vi "PKYK_TRAIL_TOKEN.vi"(1 "RFID In":string) -> (0 "PKYK?TRAIL":string)   [LabVIEW 2020]
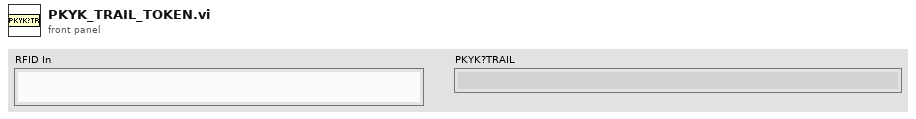
[diagram p1: front panel]
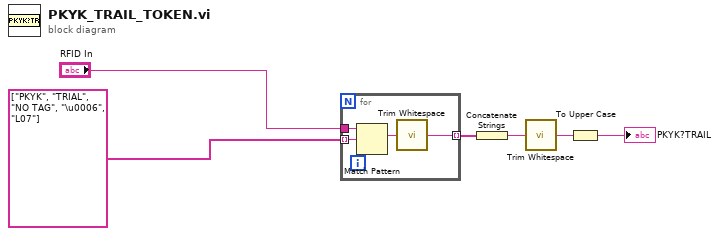
[diagram p0: block diagram]
diagram:
  n1 = for {
    tunnel: "RFID In" -> [w10]
    tunnel: [w7] -> w3 mode=indexing
    tunnel: string[] ["PKYK", "TRIAL", "NO TAG", "\u0006", "L07"] -> [w8] mode=indexing
    n2 = Match Pattern(string=w10, regular expression=w8) -> (match substring=w9:string)  [unwired: 1 in, 3 out]
    n3 = call <vilib>:"Trim Whitespace.vi"("string"=w9) -> ("trimmed string"=w7:string)  [unwired: 1 in]
  }
  n4 = Concatenate Strings(w3) -> (w4:string)
  n5 = call <vilib>:"Trim Whitespace.vi"("string"=w4) -> ("trimmed string"=w5:string)  [unwired: 1 in]
  n6 = To Upper Case(1:w5) -> (0:→"PKYK?TRAIL":string)
